vi "generate PWM Tag Lists.vi"(7 "channel":refnum<class "TBM channel.lvclass">, 8 "error in (no error)":errorcluster, 9 "Mappings in":T2 {"Line"."Parameters"."Voltage Config"."out terminal configuration (V)" items=["Default"=-1, "RSE"=10083, "Differential"=10106, "Pseudodifferential"=12529]; "Line"."Parameters"."Voltage Config"."in terminal configuration (V)" items=["Default"=-1, "RSE"=10083, "NRSE"=10078, "Differential"=10106, "Pseudodifferential"=12529]; "Line"."Parameters"."Current Config"."shunt resistor location" items=["default"=-1, "Internal"=10200, "External"=10167]; "Line"."Parameters"."Current Config"."input terminal configuration (C)" items=["default"=-1, "RSE"=10083, "NRSE"=10078, "Differential"=10106, "Pseudodifferential"=12529]; "Line"."Parameters"."RTD Config"."resistance configuration" items=["2-Wire"=2, "3-Wire"=3, "4-Wire"=4]; "Line"."Parameters"."RTD Config"."rtd type" items=["Pt3750"=12481, "Pt3851"=10071, "Pt3911"=12482, "Pt3916"=10069, "Pt3920"=10053, "Pt3928"=12483, "Custom"=10137]; "Line"."Parameters"."RTD Config"."current excitation source" items=["Internal"=10200, "External"=10167, "None"=10230]; "Line"."Parameters"."Thermocouple Config"."thermocouple type" items=["J"=10072, "K"=10073, "N"=10077, "R"=10082, "S"=10085, "T"=10086, "B"=10047, "E"=10055]; "Line"."Parameters"."Thermocouple Config"."cjc source" items=["Built-In"=10200, "Constant Value"=10116, "Channel"=10113]; "Line"."Parameters"."Strain Config"."bridge information"."strain configuration" items=["Full Bridge I"=10183, "Full Bridge II"=10184, "Full Bridge III"=10185, "Half Bridge I"=10188, "Half Bridge II"=10189, "Quarter Bridge I"=10271, "Quarter Bridge II"=10272]; "Line"."Parameters"."Strain Config"."bridge information"."voltage excitation source" items=["Internal"=10200, "External"=10167, "None"=10230]}, 10 "Measurement Type":T1, 11 "engine configuration in":refnum<class "engine configuration.lvclass">) -> (0 "Duty Cycle Index":i32=-1, 1 "Duty Cycle Array":string[](array[string]), 2 "Freq Index":i32=-1, 3 "Frequency Array":string[](array[string]))   [LabVIEW 2015, in "DAQmx Module editor node.lvclass"]
doc: "This VI will be responsible for generating the two tag lists in the editor window for PWM signals (Frequency and Duty Cycle). This is a bit complicated by the bit that the item selected in one window can't exist in the other window."
uses:
  DAQmx Module editor node.lvclass
  Mappings.ctl
  module/configuration/Line.ctl
  <vilib>/NI/Tag Bus Module Framework/channel/TBM channel.lvclass
  module/configuration/Measurement Type.ctl
  module/configuration/Parameters.ctl
  Map.ctl
  <vilib>/NI/Module Execution Interface/Engine Configuration/engine configuration.lvclass
  <vilib>/NI/Tag Bus/tag/tag descriptor.lvclass/tag descriptor.ctl
  <vilib>/NI/Tag Bus Module Framework/channel/TBM channel.lvclass/TBM channel.ctl
  <vilib>/NI/Tag Bus/tag/write data type.vi
  <vilib>/NI/Tag Bus Module Framework/channel/Write channel classification.vi
  <vilib>/NI/Tag Bus/tag/tag descriptor.lvclass
  module/configuration/Daqmx Module configuration.lvclass
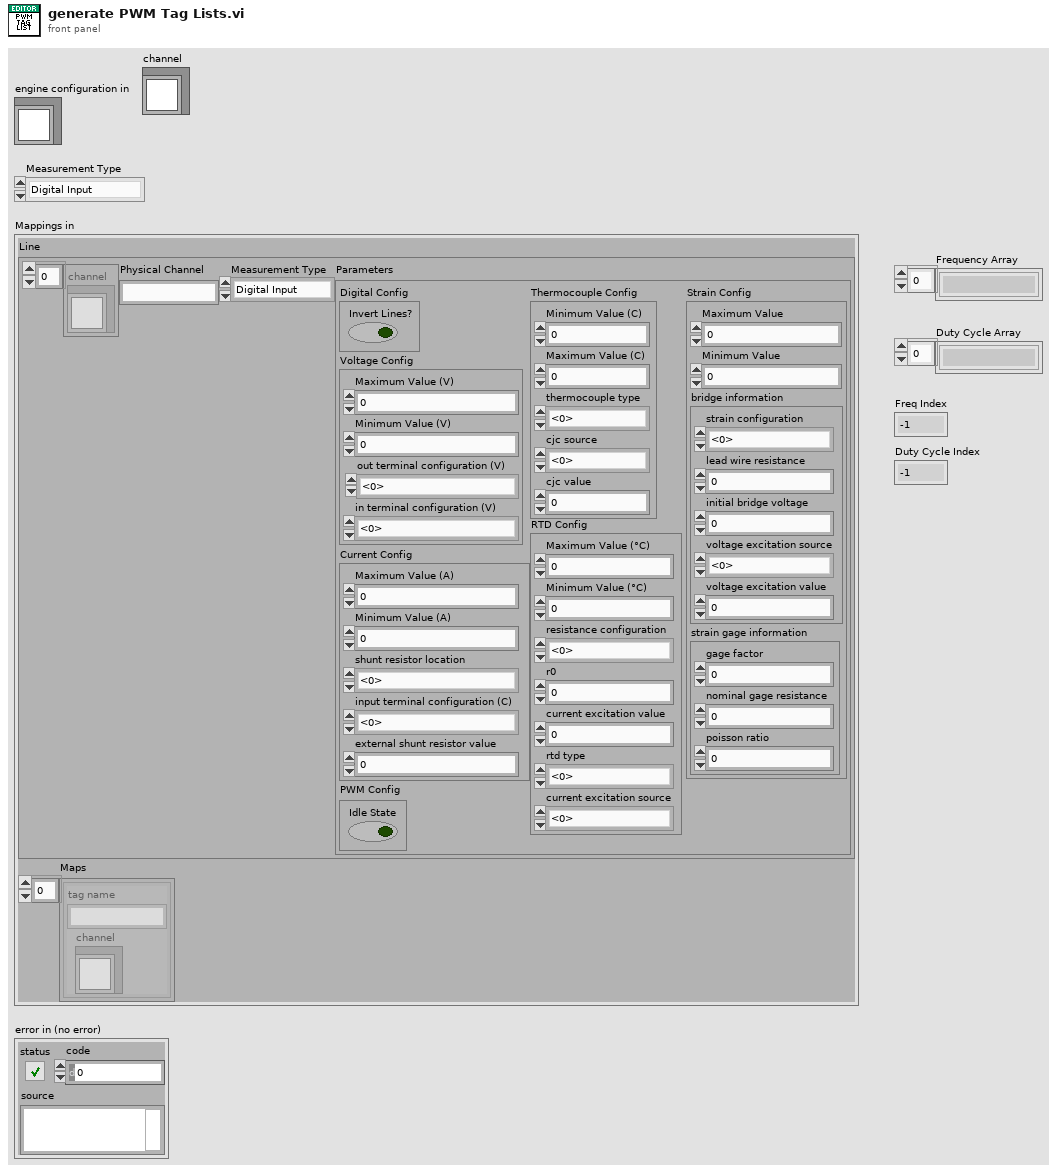
[diagram p1: front panel]
types:
  T1 = typedef "DAQmx Module Configuration.lvclass/Measurement Type.ctl" = enum16{"Digital Input", "Digital Output", "Voltage Input", "Voltage Output", "Current Input", "Current Output", "RTD", "Thermocouple", "Strain", "PWM"}
  T2 = typedef "DAQmx Module editor node.lvclass/Mappings.ctl" = cluster{"Line":T3, "Maps":T5[]}
  T3 = typedef "DAQmx Module Configuration.lvclass/Line.ctl" = cluster{"Channel Array":refnum<class "TBM channel.lvclass">[], "Physical Channel":string, "Measurement Type":T1, "Parameters":T4}
  T4 = typedef "DAQmx Module Configuration.lvclass/Parameters.ctl" = cluster{"Digital Config":cluster{"Invert Lines?":bool}, "Voltage Config":cluster{"Maximum Value (V)":dbl, "Minimum Value (V)":dbl, "in terminal configuration (V)":i32, "out terminal configuration (V)":i32}, "Current Config":cluster{"Maximum Value (A)":dbl, "Minimum Value (A)":dbl, "shunt resistor location":i32, "input terminal configuration (C)":i32, "external shunt resistor value":dbl}, "RTD Config":cluster{"Maximum Value (°C)":dbl, "Minimum Value (°C)":dbl, "resistance configuration":i32, "r0":dbl, "current excitation value":dbl, "rtd type":i32, "current excitation source":i32}, "Thermocouple Config":cluster{"Minimum Value (C)":dbl, "Maximum Value (C)":dbl, "thermocouple type":i32, "cjc source":i32, "cjc value":dbl}, "Strain Config":cluster{"Maximum Value":dbl, "Minimum Value":dbl, "bridge information":cluster{"strain configuration":i32, "lead wire resistance":dbl, "initial bridge voltage":dbl, "voltage excitation source":i32, "voltage excitation value":dbl}, "strain gage information":cluster{"gage factor":dbl, "nominal gage resistance":dbl, "poisson ratio":dbl}}, "PWM Config":cluster{"Idle State":bool}}
  T5 = typedef "DAQmx Module editor node.lvclass/Map.ctl" = cluster{"channel":refnum<class "TBM channel.lvclass">, "tag name":string}
  T6 = typedef "TBM channel.lvclass/channel classification.ctl" = enum16{"input data", "output data", "processing parameter", "processing result"}
  T7 = typedef "tag bus.lvlib/tag descriptor.lvclass/Data Type.ctl" = enum16{"Double", "Single", "I64", "I32", "I16", "I8", "U64", "U32", "U16", "U8", "Boolean", "String", "Array of Double", "Array of Single", "Array of I64", "Array of I32", "Array of I16", "Array of I8", "Array of U64", "Array of U32", "Array of U16", "Array of U8", "Array of Boolean", "Array of String"}
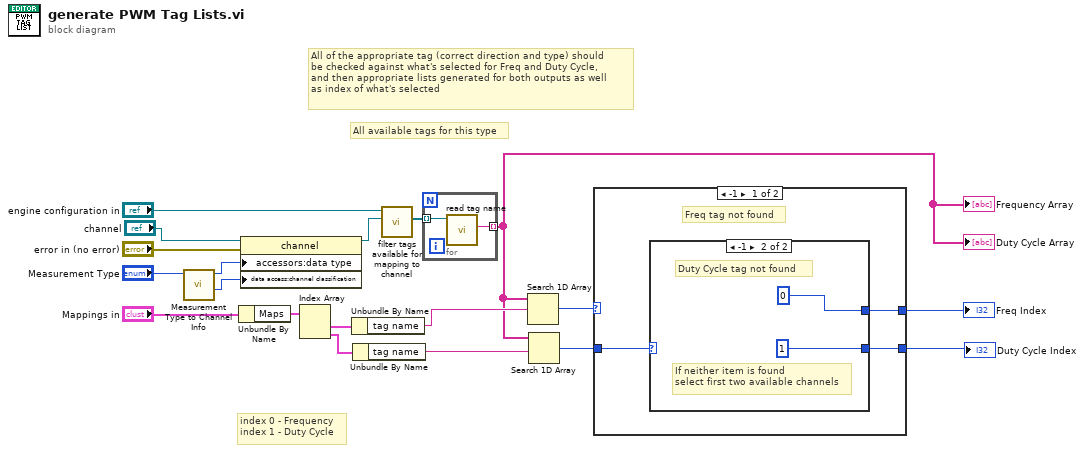
[diagram p0: block diagram]
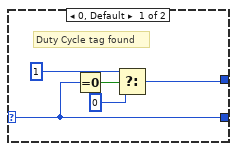
[diagram p2: hidden frame]
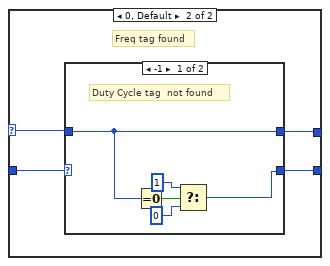
[diagram p3: hidden frame]
diagram:
  # "All of the appropriate tag (correct direction and type) should \nbe checked against what's selected for Freq and Duty Cycle, \nand then appropriate lists generated for both outputs as well\nas index of what's selected"
  # "index 0 - Frequency\nindex 1 - Duty Cycle"
  # "All available tags for this type"
  n1 = call "Measurement Type to Channel Info.vi"("Measurement Type"="Measurement Type") -> ("channel classification"=w13:T6, "Data Type"=w12:T7)  [unwired: 8 in]
  n2 = Unbundle By Name("Mappings in") -> ("Maps"=w17:T5[])
  n3 = property class="channel"(reference="channel", error in="error in (no error)", "accessors:data type"=w12, "data access:channel classification"=w13) -> (reference out=w9:refnum<class "TBM channel.lvclass">)  [unwired: 1 out]
  n4 = Index Array(array=w17) -> (element #1=w16:T5, element #2=w8:T5)  [unwired: 2 in]
  n5 = Unbundle By Name(w16) -> ("tag name"=w19:string)
  n6 = Unbundle By Name(w8) -> ("tag name"=w7:string)
  n7 = call-dynamic "filter tags available for mapping to channel.vi"("channel to map to"=w9, "engine configuration in"="engine configuration in") -> ("filtered tags"=w10:refnum<class "tag descriptor.lvclass">[])  [unwired: 8 in, 1 out]
  n8 = for {
    tunnel: w10 -> [w21] mode=indexing
    tunnel: [w20] -> w2 mode=indexing
    n9 = call <vilib>:"read tag name.vi"("system tag in"=w21) -> ("name"=w20:string)  [unwired: 8 in, 2 out]
  }
  "Frequency Array" <- w2
  "Duty Cycle Array" <- w2
  n10 = Search 1D Array(1D array=w2, element=w19) -> (index of element=w6:i32)  [unwired: 1 in]
  n11 = Search 1D Array(1D array=w2, element=w7) -> (index of element=w5:i32)  [unwired: 1 in]
  n12 = case shown="-1" w6 {
    selector: w6 -> [_ w32]
    tunnel: w5 -> [w24 w35]
    tunnel: [w23 w34] -> w4
    tunnel: [w22 w33] -> w3
    frame -1 {
      # "Freq tag not found"
      n13 = case shown="-1" w24 {
        selector: w24 -> [w26 _]
        tunnel: [w26 1 ("index of element")] -> w23
        tunnel: [w29 0 ("index of element")] -> w22
        frame 0, Default {
          # "Duty Cycle tag found"
          n14 = Equal To 0?(x=w26) -> (x = 0?=w27:bool)
          n15 = Select(t=1, s=w27, f=0) -> (s? t:f=w29:i32)
        }
        frame -1 {
          # "If neither item is found\nselect first two available channels"
          # "Duty Cycle tag not found"
        }
      }
    }
    frame 0, Default {
      # "Freq tag found"
      n16 = case shown="-1" w35 {
        selector: w35 -> [_ w41]
        tunnel: [w37 w41] -> w34
        tunnel: [w36 w42] -> w33
        tunnel: w32 -> [w36 w42]
        frame -1 {
          # "Duty Cycle tag  not found"
          n17 = Equal To 0?(x=w36) -> (x = 0?=w39:bool)
          n18 = Select(t=1, s=w39, f=0) -> (s? t:f=w37:i32)
        }
        frame Default {
          # "Need to make sure these are\nnot the same when line is added"
          # "Both found"
        }
      }
    }
  }
  "Freq Index" <- w3
  "Duty Cycle Index" <- w4
